vi "SaveConfigFile.vi"(8 "error in":errorcluster, 10 "Map":T1 {"TaskConfig"."SampleRateConfiguration"."SampleMode" items=["Finite Samples"=10178, "Continuous Samples"=10123, "Hardware Timed Single Point"=12522]}, 11 "Model Name":string) -> (0 "error out":errorcluster)   [LabVIEW 2025, in "DAQ_Module.lvlib" / "DAQ_Module.lvclass"]
uses:
  DAQ_Module.lvclass
  DAQ_Config.ctl
  DAQ_Task_Config.ctl
  DAQ_Task_Type.ctl
  2931bb75-90a3-40b0-b8f6-6a758c09f761.vi
  <vilib>/JDP Science/JSONtext/Variant to JSON Text.vi
  <vilib>/JDP Science/JSONtext/LVClass Serializer/JSONtext LVClass Serializer.lvclass
  DAQ_Module.lvclass/DAQ_Module.ctl
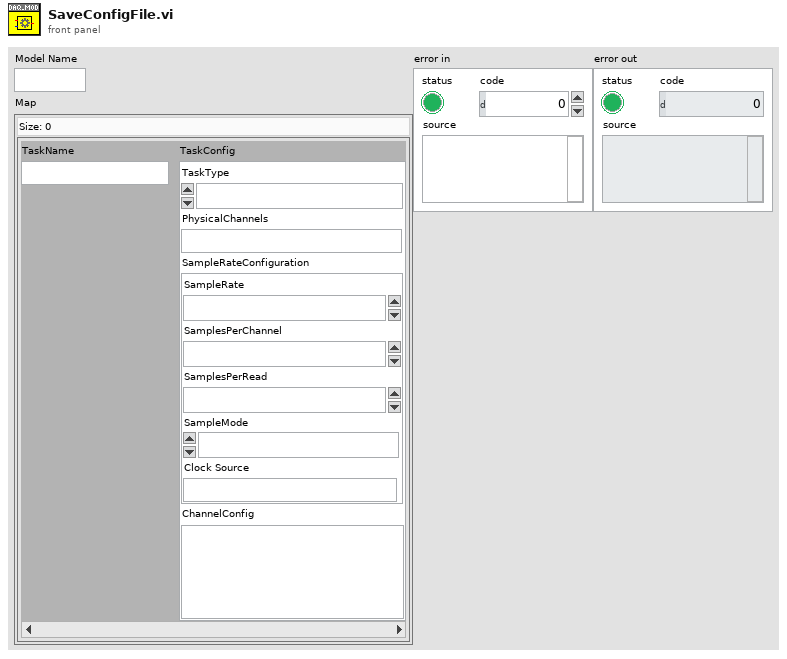
[diagram p1: front panel]
types:
  T1 = typedef "DAQ_Module.lvlib/DAQ_Module.lvclass/DAQ_Config.ctl" = map{string, T2}
  T2 = typedef "DAQ_Module.lvlib/DAQ_Module.lvclass/DAQ_Task_Config.ctl" = cluster{"TaskType":T3, "PhysicalChannels":string, "SampleRateConfiguration":cluster{"SampleRate":dbl, "SamplesPerChannel":u32, "SamplesPerRead":u32, "SampleMode":i32, "Clock Source":string}, "ChannelConfig":string}
  T3 = typedef "DAQ_Module.lvlib/DAQ_Module.lvclass/DAQ_Task_Type.ctl" = enum16{"AI", "Linear", "Angular", "AO"}
  T4 = enum16{"open", "replace", "create", "open or create", "replace or create", "replace or create with confirmation"}
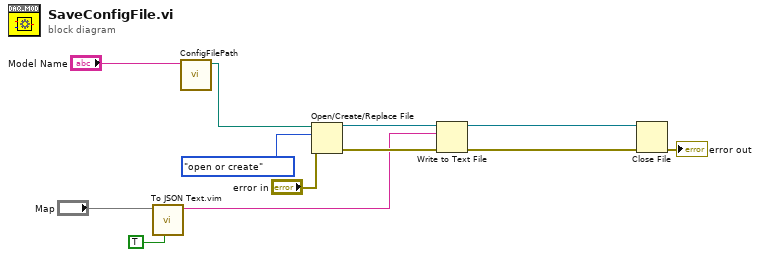
[diagram p0: block diagram]
diagram:
  n1 = call "To JSON Text.vim"("Pretty Print?"=TRUE, "Anything"="Map") -> ("<JSON>"=w1:string)  [unwired: 8 in, 1 out]
  n2 = call "ConfigFilePath.vi"("Model Name"="Model Name") -> ("appended path"=w2:path)  [unwired: 10 in]
  n3 = Open/Create/Replace File(file path (use dialog)=w2, error in="error in", operation (0:open)=T4."open or create") -> (refnum out=w8:refnum<file>, error out=w7:errorcluster)  [unwired: 3 in, 1 out]
  n4 = Write to Text File(file (use dialog)=w8, text=w1, error in=w7) -> (refnum out=w6:refnum<file>, error out=w5:errorcluster)  [unwired: 1 in, 1 out]
  n5 = Close File(refnum=w6, error in=w5) -> (error out=→"error out":errorcluster)  [unwired: 1 out]
